vi "AND.vi"(1 "b":bool, 2 "a":bool) -> (0 "x":bool)   [LabVIEW 2012]
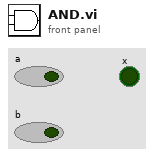
[diagram p1: front panel]
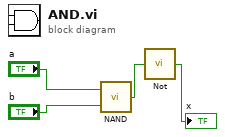
[diagram p0: block diagram]
diagram:
  n1 = call "NAND.vi"("b"="b", "a"="a") -> ("x"=w4:bool)
  n2 = call "Not.vi"("In"=w4) -> ("Out"=→"x":bool)
